vi "Lin_SelectData.vi"(7 "select？":bool, 10 "identifier":u32 format="%x", 11 "data":T1[](array[typedef]) {"payload" format="%x"; "timestamp" format="%<%.7X\n%x>T"; "type" items=["CAN Data"=0, "CAN Remote"=1, "CAN Bus Error"=2, "CAN 2.0 Data"=8, "CAN FD Data"=16, "CAN FD+BRS Data"=24, "J1939 Data"=192, "Delay"=224, "Log Trigger"=225, "Start Trigger"=226]; "identifier" format="%x"}) -> (3 "Data":T1[](array[typedef]) {"payload" format="%x"; "timestamp" format="%<%.7X\n%x>T"; "type" items=["CAN Data"=0, "CAN Remote"=1, "CAN Bus Error"=2, "CAN 2.0 Data"=8, "CAN FD Data"=16, "CAN FD+BRS Data"=24, "J1939 Data"=192, "Delay"=224, "Log Trigger"=225, "Start Trigger"=226]; "identifier" format="%x"})   [LabVIEW 2018]
uses:
  <vilib>/xnet/xnet.llb/XNET Frame CAN.ctl
  <vilib>/xnet/xnet.llb/XNET Frame Type CAN.ctl
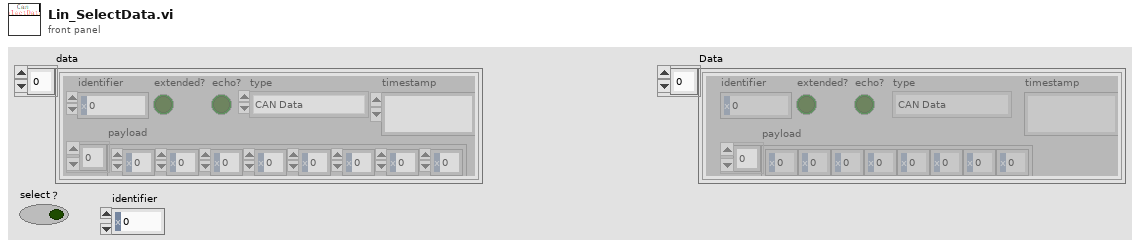
[diagram p1: front panel]
types:
  T1 = typedef "XNET Frame CAN.ctl" = cluster{"timestamp":timestamp, "payload":u8[], "identifier":u32, "type":T2, "extended?":bool, "echo?":bool}
  T2 = typedef "XNET Frame Type CAN.ctl" = u8
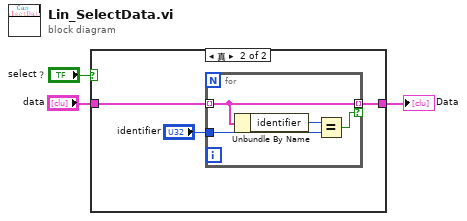
[diagram p0: block diagram]
diagram:
  n1 = case shown="真" "select？" {
    tunnel: [w4 w6] -> w3
    tunnel: "data" -> [w4 w5]
    frame False {
    }
    frame True {
      n2 = for {
        tunnel: w5 -> [w11] mode=indexing
        tunnel: "identifier" -> [w9]
        tunnel: [w11] -> w6 mode=indexing if=w8
        n3 = Unbundle By Name(w11) -> ("identifier"=w10:u32)
        n4 = Equal?(x=w10, y=w9) -> (x = y?=w8:bool)
      }
    }
  }
  "Data" <- w3
